vi "Framework Host Laptop.vi"() -> ()   [LabVIEW 2017]
uses:
  TypeDefinitions/TCP Cluster.ctl
  TypeDefinitions/TCP Commands.ctl
panel:
  out "Send":T1={"Datatype"=enum."Message", "String"="Send to sobot"}
  out "Receive":T1={"Datatype"=enum."Message", "String"="Send to sobot"}
  in  "Button 2":bool
  in  "stop":bool
  in  "Button 1":bool
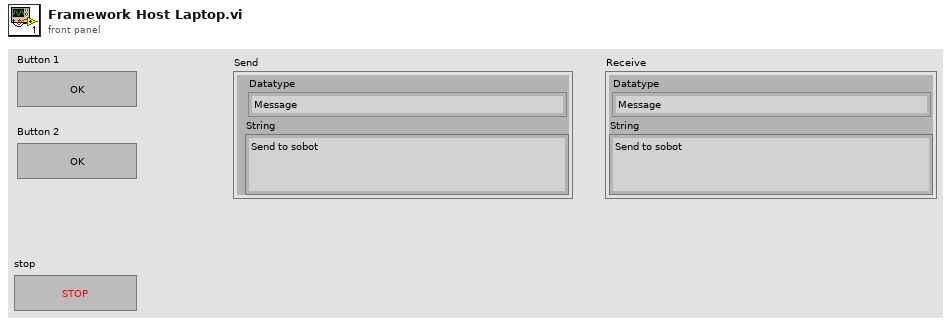
[diagram p1: front panel]
types:
  T1 = typedef "TCP Cluster.ctl" = cluster{"Datatype":T2, "String":string}
  T2 = typedef "TCP Commands.ctl" = enum16{"Message", "Stop", "Command"}
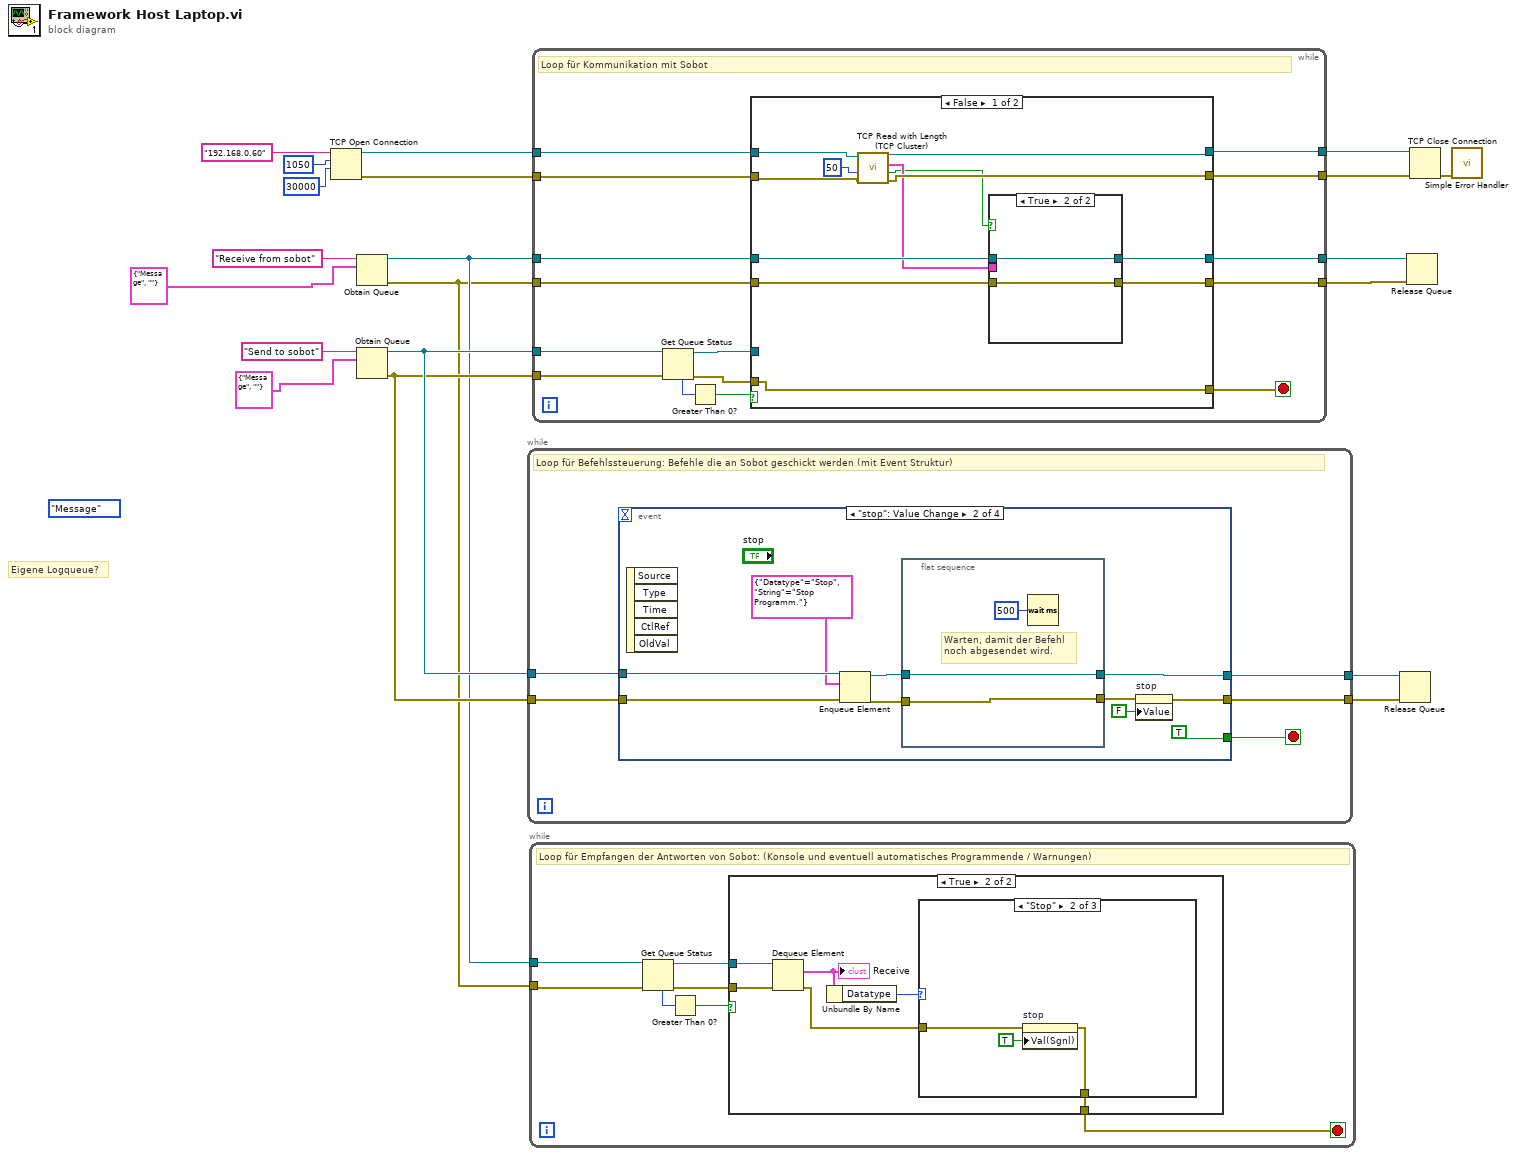
[diagram p0: block diagram]
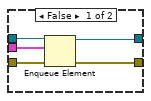
[diagram p5: hidden frame]
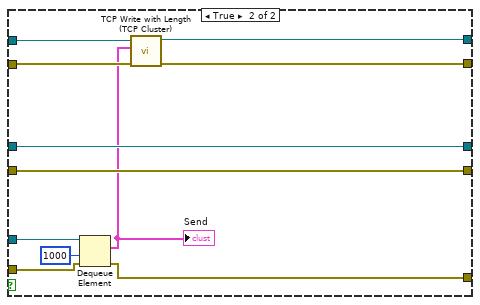
[diagram p6: hidden frame]
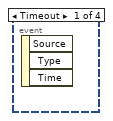
[diagram p7: hidden frame]
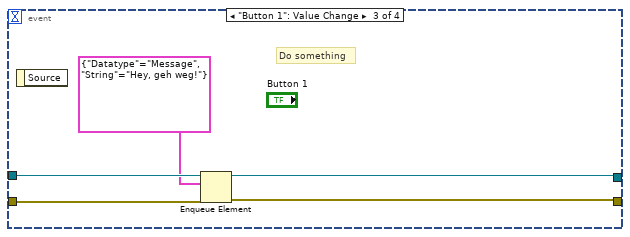
[diagram p8: hidden frame]
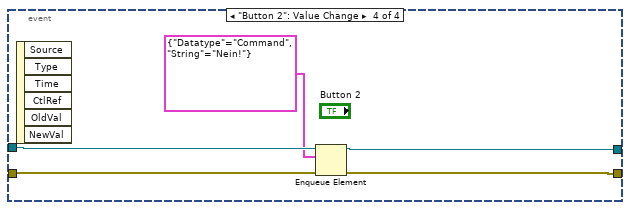
[diagram p9: hidden frame]
diagram:
  (unwired) TCP_Commands."Message"
  # "Eigene Logqueue?"
  n1 = TCP Open Connection(address="192.168.0.60", remote port or service name=u16 1050, timeout ms (60000)=30000) -> (connection ID=w12:refnum<k5>, error out=w11:errorcluster)  [unwired: 2 in]
  n2 = Obtain Queue(name (unnamed)="Receive from sobot", element data type=T1 {"Datatype"=enum."Message", "String"=""}) -> (queue out=w6:refnum<queue>, error out=w5:errorcluster)  [unwired: 3 in, 1 out]
  n3 = Obtain Queue(name (unnamed)="Send to sobot", element data type=T1 {"Datatype"=enum."Message", "String"=""}) -> (queue out=w19:refnum<queue>, error out=w16:errorcluster)  [unwired: 3 in, 1 out]
  n4 = while {
    tunnel: w19 -> [w24]
    tunnel: [w23] -> w18
    tunnel: [w22] -> w17
    tunnel: w16 -> [w21]
    stop <- w25 stop-if-true
    # "Loop für Befehlssteuerung: Befehle die an Sobot geschickt werden (mit Event Struktur)"
    n5 = event shown="[1] \"stop\": Value Change" {
      selector: _ -> [_ _ _ _]
      dyn-events: _ -> [_ _ _ _]
      timeout: _ -> [_ _ _ _]
      tunnel: [_ TRUE _ _] -> w25
      tunnel: w24 -> [_ w34 w43 w48]
      tunnel: [_ w30 w40 w47] -> w23
      tunnel: [_ w27 w41 w46] -> w22
      tunnel: w21 -> [_ w33 w42 w45]
      event Timeout {
        n6 = event-data() -> ()  [unwired: 1 in, 3 out]
      }
      event "stop": Value Change {
        n7 = event-data() -> ()  [unwired: 1 in, 5 out]
        n8 = Enqueue Element(queue=w34, element=T1 {"Datatype"=enum."Stop", "String"="Stop Programm."}, error in (no error)=w33) -> (queue out=w31:refnum<queue>, error out=w29:errorcluster)  [unwired: 1 in, 1 out]
        n9 = flat-sequence {
          tunnel: w31 -> [w38]
          tunnel: [w38] -> w30
          tunnel: [w36] -> w28
          tunnel: w29 -> [w36]
          frame #0 {
            # "Warten, damit der Befehl\nnoch abgesendet wird."
            n10 = Wait (ms)(milliseconds to wait=u32 500) -> ()  [unwired: 1 out]
          }
        }
        n11 = property on="stop" class="Bool (strict)"(error in=w28, "Value"=FALSE ("stop")) -> (error out=w27:errorcluster)  [unwired: 1 in, 1 out]
      }
      event "Button 1": Value Change {
        # "Do something"
        n12 = event-data() -> ()  [unwired: 1 in, 1 out]
        n13 = Enqueue Element(queue=w43, element=T1 {"Datatype"=enum."Message", "String"="Hey, geh weg!"}, error in (no error)=w42) -> (queue out=w40:refnum<queue>, error out=w41:errorcluster)  [unwired: 1 in, 1 out]
      }
      event "Button 2": Value Change {
        n14 = event-data() -> ()  [unwired: 1 in, 6 out]
        n15 = Enqueue Element(queue=w48, element=T1 {"Datatype"=enum."Command", "String"="Nein!"}, error in (no error)=w45) -> (queue out=w47:refnum<queue>, error out=w46:errorcluster)  [unwired: 1 in, 1 out]
      }
    }
  }
  n16 = while {
    tunnel: w6 -> [w54]
    tunnel: w5 -> [w53]
    stop <- w49 stop-if-true
    # "Loop für Empfangen der Antworten von Sobot: (Konsole und eventuell automatisches Programmende / Warnungen)"
    n17 = Get Queue Status(queue=w54, error in (no error)=w53) -> (queue out=w51:refnum<queue>, error out=w50:errorcluster, # elements in queue=w55:i32)  [unwired: 1 in, 5 out]
    n18 = Greater Than 0?(x=w55) -> (x > 0?=w52:bool)
    n19 = case shown="True" w52 {
      tunnel: w51 -> [_ w62]
      tunnel: w50 -> [w56 w61]
      tunnel: [w56 w57] -> w49
      frame False {
      }
      frame True {
        n20 = Dequeue Element(queue=w62, error in (no error)=w61) -> (element=w60:T1, error out=w58:errorcluster)  [unwired: 1 in, 2 out]
        "Receive" <- w60
        n21 = Unbundle By Name(w60) -> ("Datatype"=w59:T2)
        n22 = case shown="\"Stop\"" w59 {
          tunnel: w58 -> [w63 w65 w67]
          tunnel: [w63 w64 w67] -> w57
          frame "Message", Default {
          }
          frame "Stop" {
            n23 = property on="stop" class="Bool (strict)"(error in=w65, "Val(Sgnl)"=TRUE ("Value (Signaling)")) -> (error out=w64:errorcluster)  [unwired: 1 in, 1 out]
          }
          frame "Command" {
          }
        }
      }
    }
  }
  n24 = while {
    tunnel: w19 -> [w81]
    tunnel: w16 -> [w79]
    tunnel: w12 -> [w75]
    tunnel: w11 -> [w74]
    tunnel: [w73] -> w9
    tunnel: [w72] -> w8
    tunnel: w6 -> [w71]
    tunnel: w5 -> [w70]
    tunnel: [w69] -> w3
    tunnel: [w68] -> w4
    stop <- w82 stop-if-true
    # "Loop für Kommunikation mit Sobot"
    n25 = Get Queue Status(queue=w81, error in (no error)=w79) -> (queue out=w80:refnum<queue>, error out=w78:errorcluster, # elements in queue=w77:i32)  [unwired: 1 in, 5 out]
    n26 = Greater Than 0?(x=w77) -> (x > 0?=w76:bool)
    n27 = case shown="False" w76 {
      tunnel: [w94 w112] -> w82
      tunnel: w80 -> [_ w110]
      tunnel: w78 -> [w94 w109]
      tunnel: w75 -> [w89 w106]
      tunnel: w74 -> [w88 w105]
      tunnel: [w86 w104] -> w72
      tunnel: [w85 w103] -> w73
      tunnel: w71 -> [w93 w108]
      tunnel: w70 -> [w92 w107]
      tunnel: [w91 w108] -> w68
      tunnel: [w90 w107] -> w69
      frame False {
        n28 = call "TCP Read with Length (TCP Cluster).vi"("error in (no error)"=w88, "Timeout"=50, "connection ID"=w89) -> ("error out"=w86:errorcluster, "Timeout?"=w83:bool, "TCP Cluster"=w84:T1, "connection ID out"=w85:refnum<k5>)  [unwired: 5 in]
        n29 = case shown="True" w83 {
          tunnel: w93 -> [w99 w101]
          tunnel: w92 -> [w98 w100]
          tunnel: w84 -> [w97 _]
          tunnel: [w96 w101] -> w91
          tunnel: [w95 w100] -> w90
          frame False {
            n30 = Enqueue Element(queue=w99, element=w97, error in (no error)=w98) -> (queue out=w96:refnum<queue>, error out=w95:errorcluster)  [unwired: 1 in, 1 out]
          }
          frame True {
          }
        }
      }
      frame True {
        n31 = Dequeue Element(queue=w110, timeout in ms (-1)=1000, error in (no error)=w109) -> (element=w102:T1, error out=w112:errorcluster)  [unwired: 2 out]
        "Send" <- w102
        n32 = call "TCP Write with Length (TCP Cluster).vi"("error in (no error)"=w105, 10:w102, "connection ID"=w106) -> ("error out"=w104:errorcluster, "connection ID out"=w103:refnum<k5>)  [unwired: 7 in]
      }
    }
  }
  n33 = Release Queue(queue=w18, error in (no error)=w17) -> ()  [unwired: 1 in, 3 out]
  n34 = Release Queue(queue=w4, error in (no error)=w3) -> ()  [unwired: 1 in, 3 out]
  n35 = TCP Close Connection(connection ID=w9, error in (no error)=w8) -> (error out=w10:errorcluster)  [unwired: 1 in, 1 out]
  n36 = call <vilib>:"Simple Error Handler.vi"("error in (no error)"=w10) -> ()  [unwired: 4 in, 5 out]
